vi "onHttpPost (Buffer).vi"(8 "error in":errorcluster, 10 "httpRequest":refnum<class "httpRequest.lvclass">, 11 "advanced-http-client in":refnum<class "advanced-http-client.lvclass">) -> (0 "error out":errorcluster, 2 "httpResponse":refnum<class "httpResponse.lvclass">, 3 "advanced-http-client out":refnum<class "advanced-http-client.lvclass">)   [LabVIEW 2020, in "HttpClient.NiAdvanced.lvlib" / "advanced-http-client.lvclass"]
uses:
  advanced-http-client.lvclass
  advanced-http-client.lvclass/advanced-http-client.ctl
  <vilib>/NI/Advanced HTTP Client/Session.lvclass
  <vilib>/NI/Advanced HTTP Client/POST (Buffer).vi
  http-client-pkg/httpRequest/httpRequest.lvclass
  http-client-pkg/httpResponse/httpResponse.lvclass
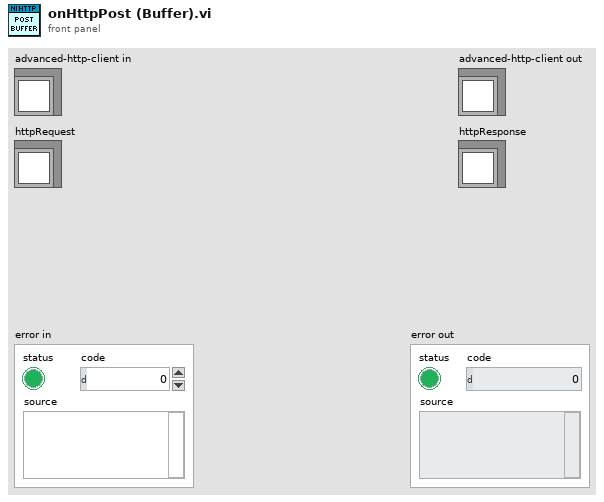
[diagram p1: front panel]
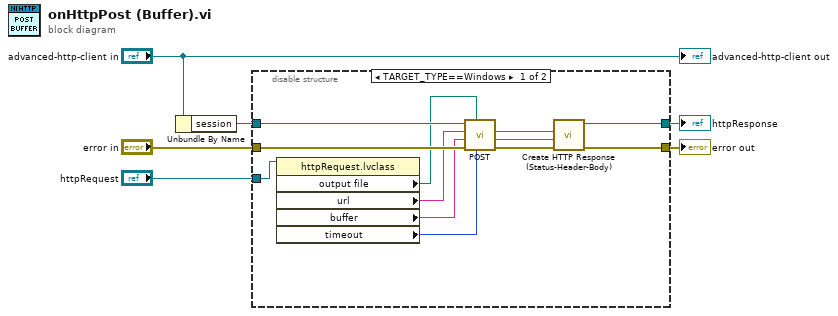
[diagram p0: block diagram]
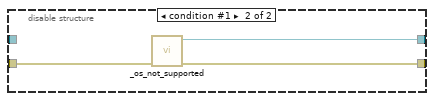
[diagram p2: hidden frame]
diagram:
  n1 = Unbundle By Name("advanced-http-client in") -> ("session"=w6:refnum<class "Session.lvclass">)
  n2 = disable-structure shown="TARGET_TYPE==Windows" {
    disable-tunnel: w6 -> [w18 _]
    disable-tunnel: "error in" -> [w17 w21]
    disable-tunnel: [w10 w20] -> w3
    disable-tunnel: "httpRequest" -> [w15 _]
    disable-tunnel: [w9 w19] -> w1
    frame condition #0 (active) {
      n3 = property class="httpRequest.lvclass"(reference=w15) -> ("output file"=w12:path, "url"=w16:string, "buffer"=w14:string, "timeout"=w13:i32)  [unwired: 1 in, 2 out]
      n4 = call-poly <vilib>:"POST.vi"("timeout"=w13, "output file"=w12, "error in"=w17, "buffer"=w14, "url"=w16, "session in"=w18) -> ("error out"=w11:errorcluster, "body"=w8:string, "headers"=w7:string)  [unwired: 1 in, 2 out]
      n5 = call "Create HTTP Response (Status-Header-Body).vi"("error in"=w11, "body"=w8, "Headers w/ status line(s)"=w7) -> ("error out"=w10:errorcluster, "httpResponse out"=w9:refnum<class "httpResponse.lvclass">)  [unwired: 7 in]
    }
    frame condition #1 {
      n6 = call "_os_not_supported.vi"("error in (no error)"=w21) -> ("error out"=w20:errorcluster, "httpResponse"=w19:refnum<class "httpResponse.lvclass">)  [unwired: 9 in]
    }
  }
  "error out" <- w3
  "httpResponse" <- w1
  "advanced-http-client out" <- "advanced-http-client in"
